vi "Send Measurement to Datalogger.vi"(8 "error in (no error)":errorcluster, 10 "Data In":dbl, 11 "Sensor in":refnum<class "Sensor.lvclass">) -> (0 "error out":errorcluster, 3 "Sensor out":refnum<class "Sensor.lvclass">)   [LabVIEW 2014]
uses:
  Sensor.lvclass
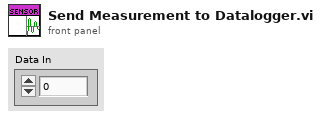
[diagram p1: front panel]
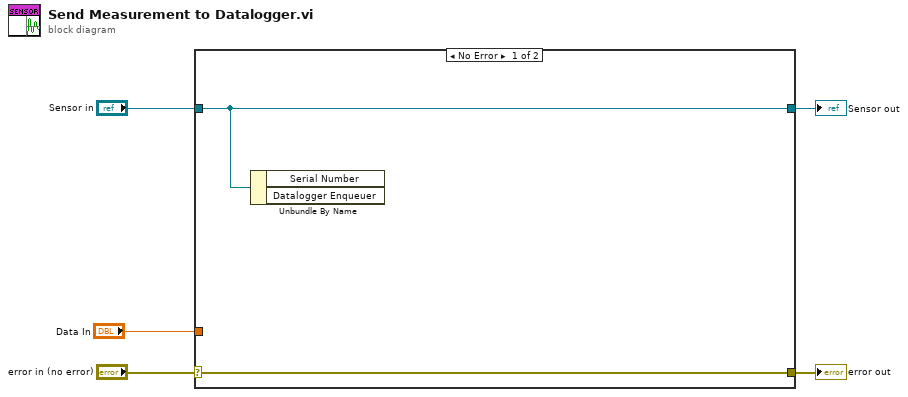
[diagram p0: block diagram]
diagram:
  n1 = case shown="No Error" "error in (no error)" {
    selector: "error in (no error)" -> [w7 w9]
    tunnel: [w7 w9] -> w4
    tunnel: [w6 w8] -> w2
    tunnel: "Sensor in" -> [w6 w8]
    tunnel: "Data In" -> [_ _]
    frame No Error {
      n2 = Unbundle By Name(w6) -> ()  [unwired: 2 out]
    }
    frame Error {
    }
  }
  "error out" <- w4
  "Sensor out" <- w2
